vi "Day15-1.vi"() -> ()   [LabVIEW 2021]
panel:
  out "XY Graph":cluster{i32[], i32[]}[](graph)
  out "Numeric":i32
  out "Array 9":i32[](array[numeric])
  out "Array 7":string[](array[string])
  out "sum 2":i32
  out "sum":i32
  out "Array 6":string[][](array[string])
  out "Array 5":string[][](array[string])
  out "min y":i32
  out "max y":i32
  out "min x":i32
  out "max x":i32
  out "Array 4":i32[](array[numeric])
  out "beacons":cluster{i32, i32}[](array[cluster])
  out "sensprs":cluster{i32, i32}[](array[cluster])
  out "sensors":i32
  out "Array":string[](array[string])
  out "array":string[][](array[string])
  # "5917380"
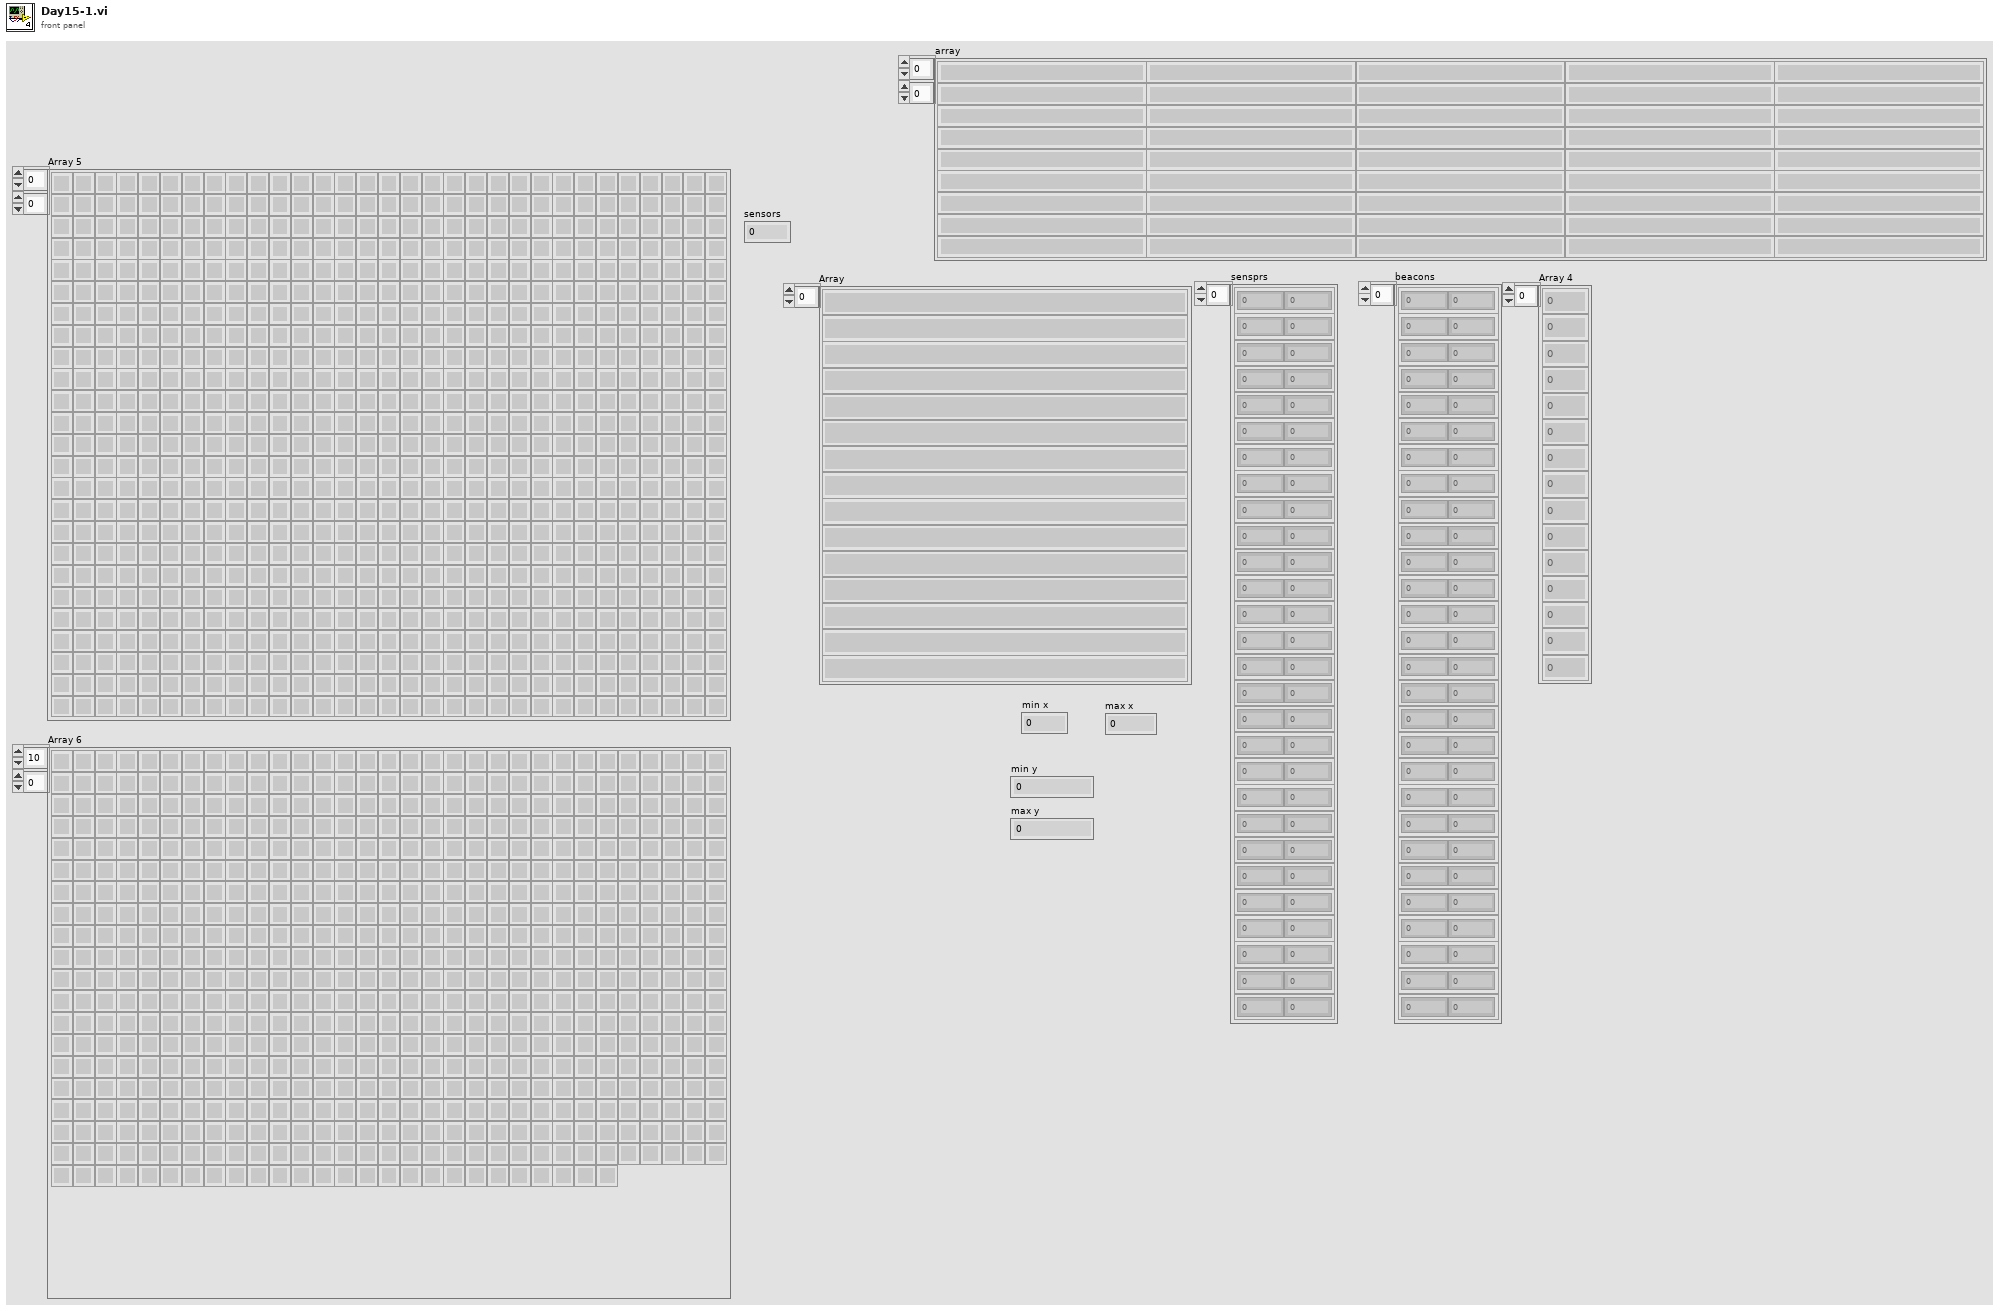
[diagram p1: front panel]
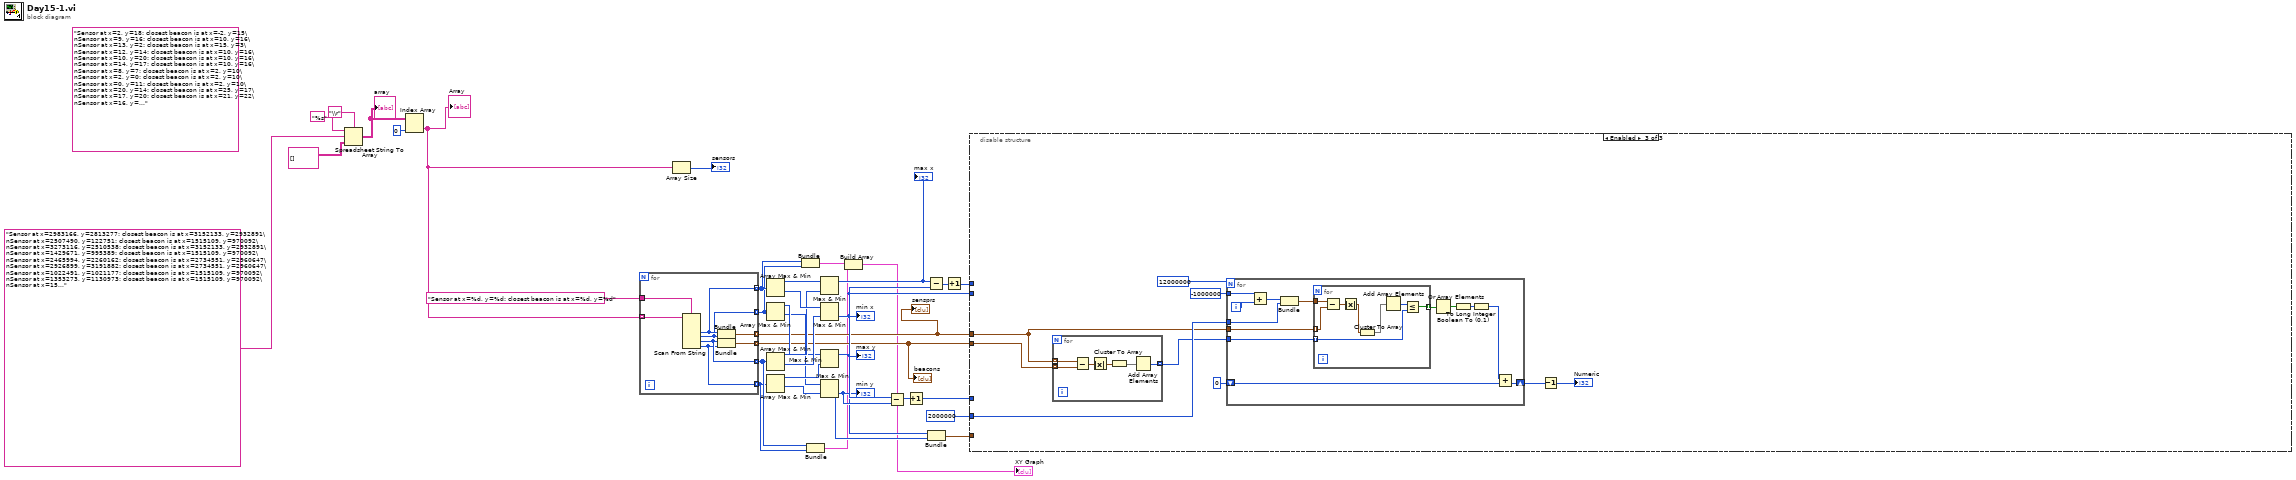
[diagram p0: block diagram]
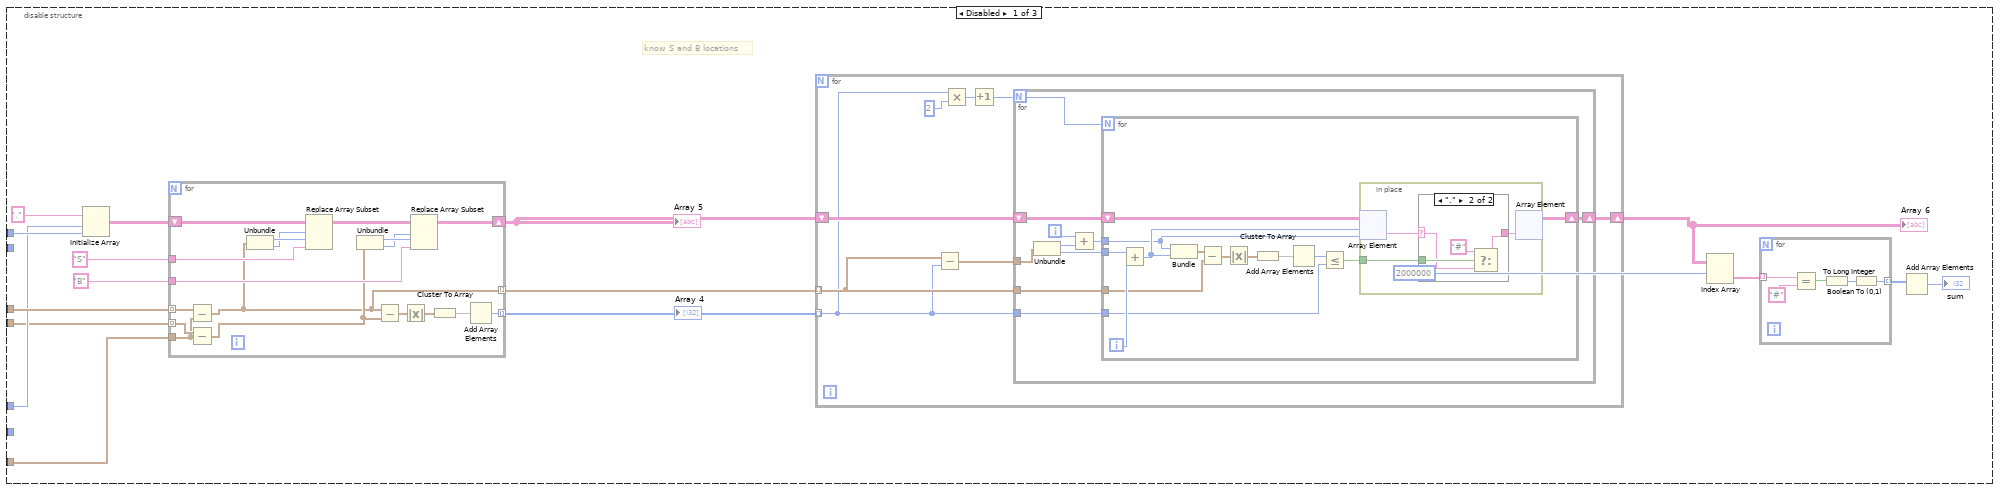
[diagram p2: hidden frame]
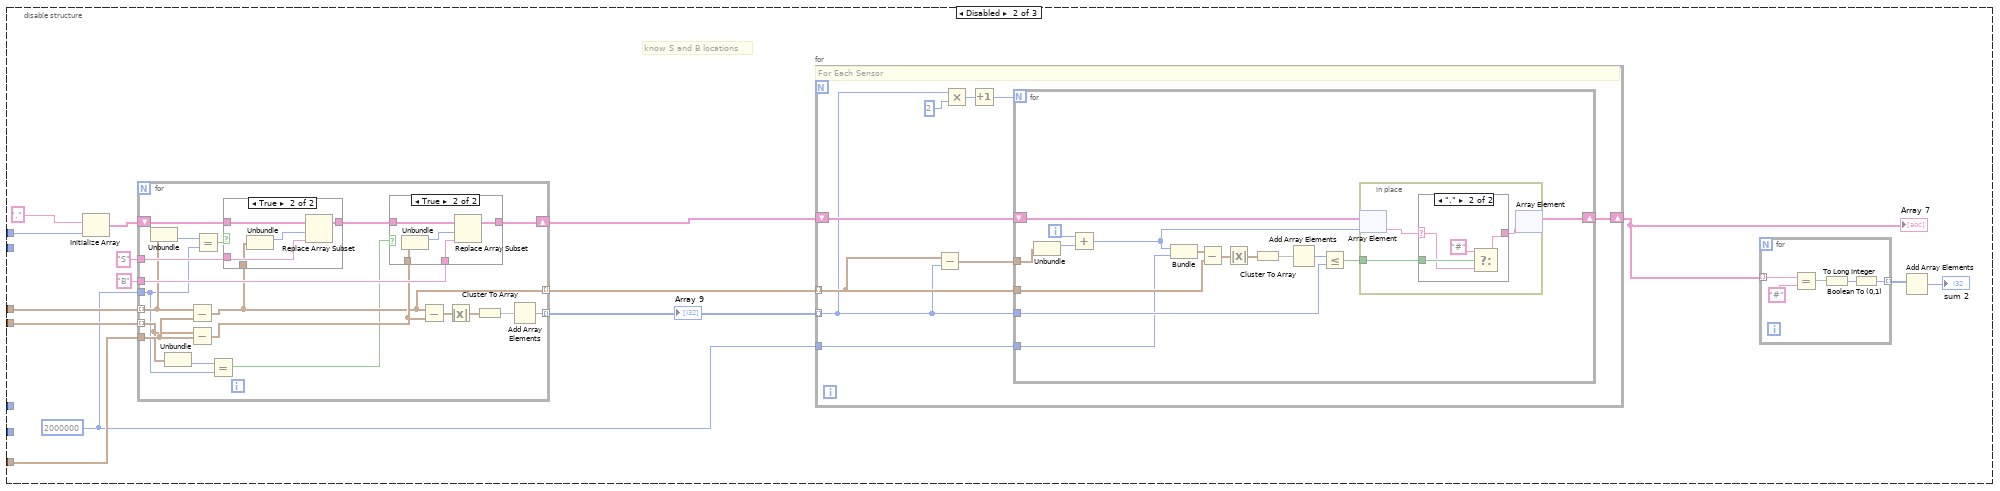
[diagram p4: hidden frame]
diagram:
  (unwired) "Sensor at x=2, y=18: closest beacon is at x=-2, y=15\nSensor at x=9, y=16: closest beacon is at x=10, y=16\nSensor at x=13, y=2: closest beacon is at x=15, y=3\nSensor at x=12, y=14: closest beacon is at x=10, y=16\nSensor at x=10, y=20: closest beacon is at x=10, y=16\nSensor at x=14, y=17: closest beacon is at x=10, y=16\nSensor at x=8, y=7: closest beacon is at x=2, y=10\nSensor at x=2, y=0: closest beacon is at x=2, y=10\nSensor at x=0, y=11: closest beacon is at x=2, y=10\nSensor at x=20, y=14: closest beacon is at x=25, y=17\nSensor at x=17, y=20: closest beacon is at x=21, y=22\nSensor at x=16, y=7: closest beacon is at x=15, y=3\nSensor at x=14, y=3: closest beacon is at x=15, y=3\nSensor at x=20, y=1: closest beacon is at x=15, y=3"
  n1 = Spreadsheet String To Array(delimiter (Tab)="\\r", format string="%s", spreadsheet string="Sensor at x=2983166, y=2813277: closest beacon is at x=3152133, y=2932891\nSensor at x=2507490, y=122751: closest beacon is at x=1515109, y=970092\nSensor at x=3273116, y=2510538: closest beacon is at x=3152133, y=2932891\nSensor at x=1429671, y=995389: closest beacon is at x=1515109, y=970092\nSensor at x=2465994, y=2260162: closest beacon is at x=2734551, y=2960647\nSensor at x=2926899, y=3191882: closest beacon is at x=2734551, y=2960647\nSensor at x=1022491, y=1021177: closest beacon is at x=1515109, y=970092\nSensor at x=1353273, y=1130973: closest beacon is at x=1515109, y=970092\nSensor at x=1565476, y=2081049: closest beacon is at x=1597979, y=2000000\nSensor at x=1841125, y=1893566: closest beacon is at x=1597979, y=2000000\nSensor at x=99988, y=71317: closest beacon is at x=86583, y=-1649857\nSensor at x=3080600, y=3984582: closest beacon is at x=3175561, y=4138060\nSensor at x=3942770, y=3002123: closest beacon is at x=3724687, y=3294321\nSensor at x=1572920, y=2031447: closest beacon is at x=1597979, y=2000000\nSensor at x=218329, y=1882777: closest beacon is at x=1597979, y=2000000\nSensor at x=1401723, y=1460526: closest beacon is at x=1515109, y=970092\nSensor at x=2114094, y=985978: closest beacon is at x=1515109, y=970092\nSensor at x=3358586, y=3171857: closest beacon is at x=3152133, y=2932891\nSensor at x=1226284, y=3662922: closest beacon is at x=2514367, y=3218259\nSensor at x=3486366, y=3717867: closest beacon is at x=3724687, y=3294321\nSensor at x=1271873, y=831354: closest beacon is at x=1515109, y=970092\nSensor at x=3568311, y=1566400: closest beacon is at x=3152133, y=2932891\nSensor at x=3831960, y=3146611: closest beacon is at x=3724687, y=3294321\nSensor at x=2505534, y=3196726: closest beacon is at x=2514367, y=3218259\nSensor at x=2736967, y=3632098: closest beacon is at x=2514367, y=3218259\nSensor at x=3963402, y=3944423: closest beacon is at x=3724687, y=3294321\nSensor at x=1483115, y=2119639: closest beacon is at x=1597979, y=2000000", array type (2D Dbl)=string[][] []) -> (array=w32:string[][])
  "array" <- w32
  n2 = Index Array(array=w32, index (col)=0 ("disabled index (col)")) -> (element=w30:string[])  [unwired: 1 in]
  "Array" <- w30
  n3 = for {
    tunnel: w30 -> [w44] mode=indexing
    tunnel: "Sensor at x=%d, y=%d: closest beacon is at x=%d, y=%d" ("format string") -> [w43]
    tunnel: [w42] -> w8 mode=indexing
    tunnel: [w41] -> w9 mode=indexing
    tunnel: [w40] -> w5 mode=indexing
    tunnel: [w39] -> w4 mode=indexing
    tunnel: [w38] -> w7 mode=indexing
    tunnel: [w37] -> w6 mode=indexing
    n4 = Scan From String(format string=w43, input string=w44) -> (output 1=w40:i32, output 2=w39:i32, output 3=w38:i32, output 4=w37:i32)  [unwired: 6 in, 3 out]
    n5 = Bundle(w40, w39) -> (w42:cluster{i32, i32})  [unwired: 1 in]
    n6 = Bundle(w38, w37) -> (w41:cluster{i32, i32})  [unwired: 1 in]
  }
  "sensprs" <- w8
  "beacons" <- w9
  n7 = Array Size(array=w30) -> (size(s)=→"sensors":i32)
  n8 = Array Max & Min(array=w5) -> (max value=w28:i32, min value=w27:i32)  [unwired: 2 out]
  n9 = Array Max & Min(array=w4) -> (max value=w24:i32, min value=w21:i32)  [unwired: 2 out]
  n10 = Array Max & Min(array=w7) -> (max value=w26:i32, min value=w25:i32)  [unwired: 2 out]
  n11 = Array Max & Min(array=w6) -> (max value=w23:i32, min value=w22:i32)  [unwired: 2 out]
  n12 = Bundle(w5, w4) -> (w3:cluster{i32[], i32[]})  [unwired: 1 in]
  n13 = Bundle(w7, w6) -> (w2:cluster{i32[], i32[]})  [unwired: 1 in]
  n14 = Max & Min(x=w28, y=w26) -> (max(x,y)=w17:i32)  [unwired: 1 out]
  "max x" <- w17
  n15 = Max & Min(x=w27, y=w25) -> (min(x,y)=w11:i32)  [unwired: 1 out]
  "min x" <- w11
  n16 = Max & Min(x=w24, y=w23) -> (max(x,y)=w20:i32)  [unwired: 1 out]
  "max y" <- w20
  n17 = Max & Min(x=w21, y=w22) -> (min(x,y)=w14:i32)  [unwired: 1 out]
  "min y" <- w14
  n18 = Build Array(w3, w2) -> (→"XY Graph":cluster{i32[], i32[]}[])
  n19 = Subtract(x=w20, y=w14) -> (x-y=w19:i32)
  n20 = Increment(x=w19) -> (x+1=w15:i32)
  n21 = Subtract(x=w17, y=w11) -> (x-y=w18:i32)
  n22 = Bundle(w11, w14) -> (w13:cluster{i32, i32})  [unwired: 1 in]
  n23 = Increment(x=w18) -> (x+1=w16:i32)
  n24 = disable-structure shown="Enabled" {
    disable-tunnel: w8 -> [w61 w139 w214]
    disable-tunnel: w16 -> [w60 w138 _]
    disable-tunnel: w15 -> [w59 _ _]
    disable-tunnel: w9 -> [w57 w136 w216]
    disable-tunnel: w13 -> [w45 w126 _]
    disable-tunnel: 2000000 ("index (row)") -> [_ _ w215]
    disable-tunnel: w11 -> [_ _ _]
    frame Disabled {
      # "know S and B locations"
      n25 = Initialize Array("." ("x+1"), w59, w60) -> (w56:string[][])
      n26 = for {
        tunnel: w61 -> [w113] mode=indexing
        tunnel: w57 -> [w115] mode=indexing
        tunnel: [w121] -> w52 mode=indexing
        shift-right: [w116] -> w53
        shift-left: w56 -> [w120]
        tunnel: "B" ("x+1") -> [w117]
        tunnel: "S" ("x+1") -> [w119]
        tunnel: w45 -> [w114]
        tunnel: [w107] -> w51 mode=indexing
        n27 = Subtract(x=w113, y=w114) -> (x-y=w107:cluster{i32, i32})
        n28 = Subtract(x=w115, y=w114) -> (x-y=w108:cluster{i32, i32})
        n29 = Unbundle(w107) -> (w112:i32, w111:i32)
        n30 = Replace Array Subset(array=w120, new element=w119, index (row)=w111, index (col)=w112) -> (w118:string[][])
        n31 = Unbundle(w108) -> (w110:i32, w109:i32)
        n32 = Subtract(x=w107, y=w108) -> (x-y=w124:cluster{i32, i32})
        n33 = Absolute Value(x=w124) -> (abs(x)=w123:cluster{i32, i32})
        n34 = Replace Array Subset(array=w118, new element=w117, index (row)=w109, index (col)=w110) -> (w116:string[][])
        n35 = Cluster To Array(cluster=w123) -> (array=w122:i32[])
        n36 = Add Array Elements(numeric array=w122) -> (sum=w121:i32)
      }
      "Array 4" <- w52
      "Array 5" <- w53
      n37 = for {
        shift-right: [w73] -> w49
        shift-left: w53 -> [w74]
        tunnel: w52 -> [w68] mode=indexing
        tunnel: w51 -> [w69] mode=indexing
        n38 = Subtract(x=w69, y=w68) -> (x-y=w67:cluster{i32, i32})
        n39 = Multiply(x=w68, y=2) -> (x*y=w71:i32)
        n40 = Increment(x=w71) -> (x+1=w70:i32)
        n41 = for {
          N: w70 -> [w80]
          shift-right: [w81] -> w73
          shift-left: w74 -> [w84]
          tunnel: w69 -> [w83]
          tunnel: w68 -> [w82]
          tunnel: w67 -> [w79]
          i -> [w77]
          n42 = Unbundle(w79) -> (w78:i32, w76:i32)
          n43 = Add(x=w77, y=w78) -> (x+y=w75:i32)
          n44 = for {
            N: w80 -> [_]
            shift-right: [w85] -> w81
            shift-left: w84 -> [w89]
            tunnel: w83 -> [w93]
            tunnel: w82 -> [w90]
            tunnel: w76 -> [w98]
            tunnel: w75 -> [w87]
            i -> [w97]
            n45 = Add(x=w98, y=w97) -> (x+y=w88:i32)
            n46 = Bundle(w87, w88) -> (w92:cluster{i32, i32})  [unwired: 1 in]
            n47 = Subtract(x=w92, y=w93) -> (x-y=w96:cluster{i32, i32})
            n48 = Absolute Value(x=w96) -> (abs(x)=w95:cluster{i32, i32})
            n49 = Cluster To Array(cluster=w95) -> (array=w94:i32[])
            n50 = Add Array Elements(numeric array=w94) -> (sum=w91:i32)
            n51 = Less Or Equal?(x=w91, y=w90) -> (x <= y?=w86:bool)
            n52 = in-place {
              in-place-border: w86 -> [w99]
              n53 = in-place-array #1(w89, w88, w87) -> (w101:string)
              n54 = case shown="\".\"" w101 {
                selector: w101 -> [w102 w105]
                tunnel: [w102 w103] -> w100
                tunnel: w99 -> [_ w106]
                frame Default {
                }
                frame "." {
                  n55 = Select(t="#" ("x+1"), s=w106, f=w105) -> (s? t:f=w103:string)
                }
              }
              n56 = in-place-array #1(w100) -> (w85:string[][])  [unwired: 2 out]
            }
          }
        }
      }
      "Array 6" <- w49
      n57 = Index Array(array=w49, index (row)=2000000) -> (element=w48:string[])  [unwired: 1 in]
      n58 = for {
        tunnel: w48 -> [w66] mode=indexing
        tunnel: [w62] -> w47 mode=indexing
        n59 = Equal?(x=w66, y="#" ("x+1")) -> (x = y?=w64:bool)
        n60 = Boolean To (0,1)(Boolean=w64) -> (0, 1=w63:i16)
        n61 = To Long Integer(number=w63) -> (32bit integer=w62:i32)
      }
      n62 = Add Array Elements(numeric array=w47) -> (sum=→"sum":i32)
    }
    frame Disabled {
      w125 = 2000000 ("index (row)")
      # "know S and B locations"
      n63 = Initialize Array("." ("x+1"), w138) -> (w135:string[])
      n64 = for {
        tunnel: w139 -> [w183] mode=indexing
        tunnel: w136 -> [w179] mode=indexing
        tunnel: [w192] -> w131 mode=indexing
        shift-right: [w187] -> w132
        shift-left: w135 -> [w191]
        tunnel: "B" ("x+1") -> [w188]
        tunnel: "S" ("x+1") -> [w190]
        tunnel: w126 -> [w186]
        tunnel: [w184] -> w130 mode=indexing
        tunnel: w125 -> [w178]
        n65 = Unbundle(w183) -> (w182:i32)  [unwired: 1 out]
        n66 = Unbundle(w179) -> (w180:i32)  [unwired: 1 out]
        n67 = Subtract(x=w183, y=w186) -> (x-y=w184:cluster{i32, i32})
        n68 = Subtract(x=w179, y=w186) -> (x-y=w185:cluster{i32, i32})
        n69 = Equal?(x=w182, y=w178) -> (x = y?=w181:bool)
        n70 = Equal?(x=w180, y=w178) -> (x = y?=w177:bool)
        n71 = case shown="True" w181 {
          tunnel: w191 -> [w202 w207]
          tunnel: w190 -> [_ w206]
          tunnel: [w202 w205] -> w189
          tunnel: w184 -> [_ w204]
          frame False {
          }
          frame True {
            n72 = Unbundle(w204) -> (w203:i32)  [unwired: 1 out]
            n73 = Replace Array Subset(array=w207, new element=w206, index=w203) -> (w205:string[])
          }
        }
        n74 = case shown="True" w177 {
          tunnel: w189 -> [w196 w201]
          tunnel: w188 -> [_ w200]
          tunnel: [w196 w199] -> w187
          tunnel: w185 -> [_ w198]
          frame False {
          }
          frame True {
            n75 = Unbundle(w198) -> (w197:i32)  [unwired: 1 out]
            n76 = Replace Array Subset(array=w201, new element=w200, index=w197) -> (w199:string[])
          }
        }
        n77 = Subtract(x=w184, y=w185) -> (x-y=w195:cluster{i32, i32})
        n78 = Absolute Value(x=w195) -> (abs(x)=w194:cluster{i32, i32})
        n79 = Cluster To Array(cluster=w194) -> (array=w193:i32[])
        n80 = Add Array Elements(numeric array=w193) -> (sum=w192:i32)
      }
      "Array 9" <- w131
      n81 = for {
        shift-right: [w152] -> w129
        shift-left: w132 -> [w153]
        tunnel: w131 -> [w147] mode=indexing
        tunnel: w130 -> [w148] mode=indexing
        tunnel: w125 -> [w145]
        # "For Each Sensor"
        n82 = Subtract(x=w148, y=w147) -> (x-y=w146:cluster{i32, i32})
        n83 = Multiply(x=w147, y=2) -> (x*y=w150:i32)
        n84 = Increment(x=w150) -> (x+1=w149:i32)
        n85 = for {
          N: w149 -> [_]
          shift-right: [w165] -> w152
          shift-left: w153 -> [w168]
          tunnel: w148 -> [w167]
          tunnel: w147 -> [w166]
          tunnel: w146 -> [w164]
          tunnel: w145 -> [w154]
          i -> [w162]
          n86 = Unbundle(w164) -> (w163:i32)  [unwired: 1 out]
          n87 = Add(x=w162, y=w163) -> (x+y=w155:i32)
          n88 = Bundle(w155, "index (row)"=w154) -> (w158:cluster{i32, "index (row)":i32})  [unwired: 1 in]
          n89 = Subtract(x=w158, y=w167) -> (x-y=w161:cluster{i32, i32})
          n90 = Absolute Value(x=w161) -> (abs(x)=w160:cluster{i32, i32})
          n91 = Cluster To Array(cluster=w160) -> (array=w159:i32[])
          n92 = Add Array Elements(numeric array=w159) -> (sum=w157:i32)
          n93 = Less Or Equal?(x=w157, y=w166) -> (x <= y?=w156:bool)
          n94 = in-place {
            in-place-border: w156 -> [w169]
            n95 = in-place-array #2(w168, w155) -> (w171:string)
            n96 = case shown="\".\"" w171 {
              selector: w171 -> [w172 w175]
              tunnel: [w172 w173] -> w170
              tunnel: w169 -> [_ w176]
              frame Default {
              }
              frame "." {
                n97 = Select(t="#" ("x+1"), s=w176, f=w175) -> (s? t:f=w173:string)
              }
            }
            n98 = in-place-array #2(w170) -> (w165:string[])  [unwired: 1 out]
          }
        }
      }
      "Array 7" <- w129
      n99 = for {
        tunnel: w129 -> [w144] mode=indexing
        tunnel: [w140] -> w128 mode=indexing
        n100 = Equal?(x=w144, y="#" ("x+1")) -> (x = y?=w142:bool)
        n101 = Boolean To (0,1)(Boolean=w142) -> (0, 1=w141:i16)
        n102 = To Long Integer(number=w141) -> (32bit integer=w140:i32)
      }
      n103 = Add Array Elements(numeric array=w128) -> (sum=→"sum 2":i32)
    }
    frame Enabled {
      n104 = for {
        tunnel: w214 -> [w240] mode=indexing
        tunnel: w216 -> [w239] mode=indexing
        tunnel: [w238] -> w213 mode=indexing
        n105 = Subtract(x=w240, y=w239) -> (x-y=w243:cluster{i32, i32})
        n106 = Absolute Value(x=w243) -> (abs(x)=w242:cluster{i32, i32})
        n107 = Cluster To Array(cluster=w242) -> (array=w241:i32[])
        n108 = Add Array Elements(numeric array=w241) -> (sum=w238:i32)
      }
      n109 = for {
        N: 12000000 -> [_]
        tunnel: -1000000 -> [w229]
        tunnel: w215 -> [w226]
        tunnel: w214 -> [w224]
        tunnel: w213 -> [w223]
        shift-right: [w219] -> w211
        shift-left: 0 -> [w218]
        i -> [w228]
        n110 = Add(x=w229, y=w228) -> (x+y=w227:i32)
        n111 = Bundle(w227, "index (row)"=w226) -> (w225:cluster{i32, "index (row)":i32})  [unwired: 1 in]
        n112 = for {
          tunnel: w225 -> [w234]
          tunnel: w224 -> [w233] mode=indexing
          tunnel: w223 -> [w231] mode=indexing
          tunnel: [w230] -> w222 mode=indexing
          n113 = Subtract(x=w234, y=w233) -> (x-y=w235:cluster{i32, i32})
          n114 = Absolute Value(x=w235) -> (abs(x)=w236:cluster{i32, i32})
          n115 = Cluster To Array(cluster=w236) -> (array=w237:i32[])
          n116 = Add Array Elements(numeric array=w237) -> (sum=w232:i32)
          n117 = Less Or Equal?(x=w232, y=w231) -> (x <= y?=w230:bool)
        }
        n118 = Or Array Elements(Boolean array=w222) -> (logical OR=w221:bool)
        n119 = Boolean To (0,1)(Boolean=w221) -> (0, 1=w220:i16)
        n120 = To Long Integer(number=w220) -> (32bit integer=w217:i32)
        n121 = Add(x=w217, y=w218) -> (x+y=w219:i32)
      }
      n122 = Decrement(x=w211) -> (x-1=→"Numeric":i32)
    }
  }
